vi "Get Model Info - from DLL.vi"(0 "Model Filepaths":path[](array[path]), 4 "Models":string[](array[string]), 5 "Error (in)":errorcluster) -> (14 "DLL Inports":string[](array[string]), 15 "DLL Outports":string[](array[string]), 16 "DLL Parameters":string[](array[string]), 17 "DLL Signals":string[](array[string]), 19 "Error (out)":errorcluster)   [LabVIEW 2016]
uses:
  <vilib>/Model Interface Toolkit/Get Inport Paths.vi
  <vilib>/Model Interface Toolkit/Get Outport Paths.vi
  <vilib>/Model Interface Toolkit/Get Parameter Paths.vi
  <vilib>/Model Interface Toolkit/Get Signal Paths.vi
  <vilib>/Model Interface Toolkit/Model Interface Toolkit.lvclass
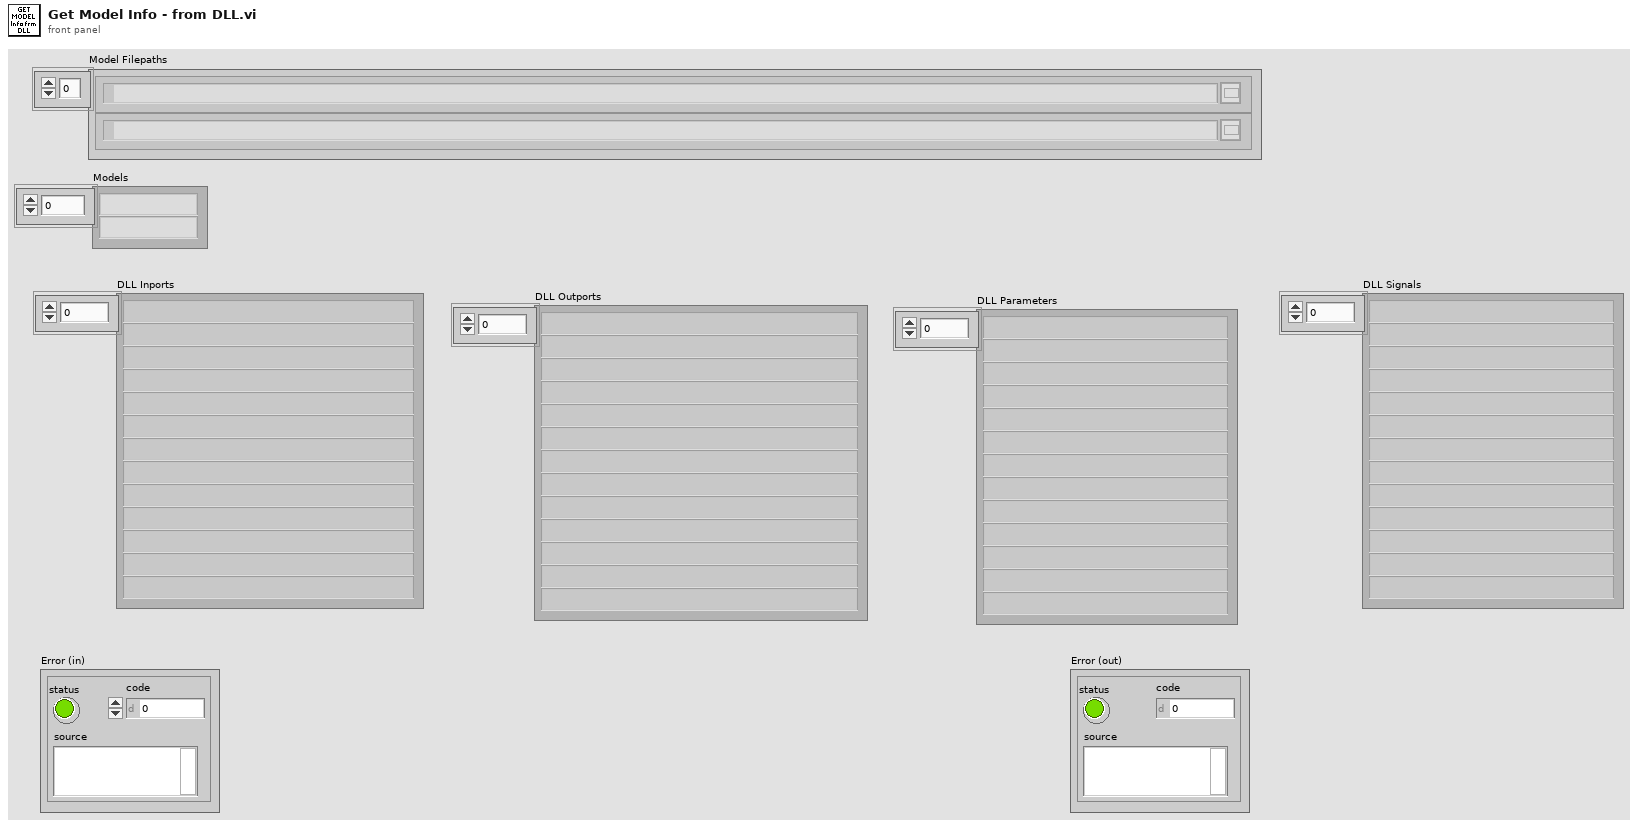
[diagram p1: front panel]
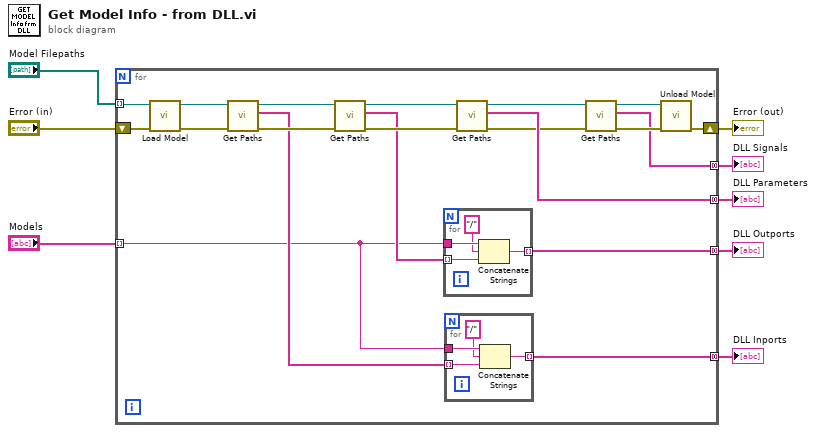
[diagram p0: block diagram]
diagram:
  n1 = for {
    tunnel: "Model Filepaths" -> [w21] mode=indexing
    shift-right: [w20] -> w7
    shift-left: "Error (in)" -> [w22]
    tunnel: [w19] -> w6 mode=concatenating
    tunnel: [w17] -> w5 mode=concatenating
    tunnel: [w15] -> w4 mode=concatenating
    tunnel: "Models" -> [w14] mode=indexing
    tunnel: [w9] -> w1 mode=concatenating
    n2 = call <vilib>:"Load Model.vi"("error in (no error)"=w22, "Model Path"=w21) -> ("error out"=w25:errorcluster, "Model out"=w26:refnum<class "Model Interface Toolkit.lvclass">)  [unwired: 8 in]
    n3 = call-poly <vilib>:"Get Paths.vi"("error in (no error)"=w25, "Model in"=w26) -> ("error out"=w24:errorcluster, "Inport Paths"=w16:string[], "Model out"=w27:refnum<class "Model Interface Toolkit.lvclass">)  [unwired: 7 in]
    n4 = call-poly <vilib>:"Get Paths.vi"("error in (no error)"=w24, "Model in"=w27) -> ("error out"=w23:errorcluster, "Outport Paths"=w18:string[], "Model out"=w28:refnum<class "Model Interface Toolkit.lvclass">)  [unwired: 7 in]
    n5 = for {
      tunnel: w14 -> [w36]
      tunnel: w18 -> [w35] mode=indexing
      tunnel: [w33] -> w17 mode=indexing
      n6 = Concatenate Strings(w36, "/" ("string"), w35) -> (w33:string)
    }
    n7 = for {
      tunnel: w14 -> [w32]
      tunnel: w16 -> [w31] mode=indexing
      tunnel: [w29] -> w15 mode=indexing
      n8 = Concatenate Strings(w32, "/" ("string"), w31) -> (w29:string)
    }
    n9 = call-poly <vilib>:"Get Paths.vi"("error in"=w23, "Model in"=w28) -> ("error out"=w13:errorcluster, "Parameter Paths"=w19:string[], "Model out"=w11:refnum<class "Model Interface Toolkit.lvclass">)  [unwired: 7 in]
    n10 = call-poly <vilib>:"Get Paths.vi"("error in"=w13, "Model in"=w11) -> ("error out"=w12:errorcluster, "Signal Paths"=w9:string[], "Model out"=w10:refnum<class "Model Interface Toolkit.lvclass">)  [unwired: 7 in]
    n11 = call <vilib>:"Unload Model.vi"("error in (no error)"=w12, "Model in"=w10) -> ("error out"=w20:errorcluster)  [unwired: 9 in]
  }
  "DLL Parameters" <- w6
  "Error (out)" <- w7
  "DLL Inports" <- w4
  "DLL Outports" <- w5
  "DLL Signals" <- w1
